vi "ArmTangentPath.vi"(1 "Radius":dbl, 2 "EndPoint":T2, 3 "PathIn":T1[](array[typedef])) -> (0 "PathOut":T1[](array[typedef]))   [LabVIEW 2018]
uses:
  TypeDefs/ArmCoordinate.ctl
  ArgosLib/Path Planning/TypeDefs/Point2D.ctl
  ArgosLib/ArgosLib.lvlib
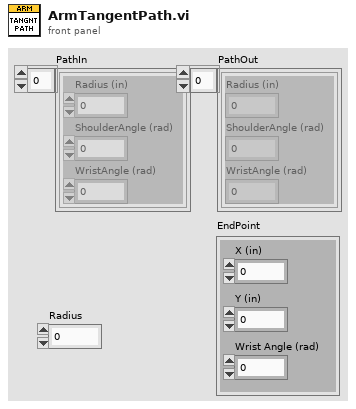
[diagram p1: front panel]
types:
  T1 = typedef "ArmCoordinate.ctl" = cluster{"Radius (in)":dbl, "ShoulderAngle (rad)":dbl, "WristAngle (rad)":dbl}
  T2 = typedef "ArgosLib.lvlib/Point2D.ctl" = cluster{"X (in)":dbl, "Y (in)":dbl, "Wrist Angle (rad)":dbl}
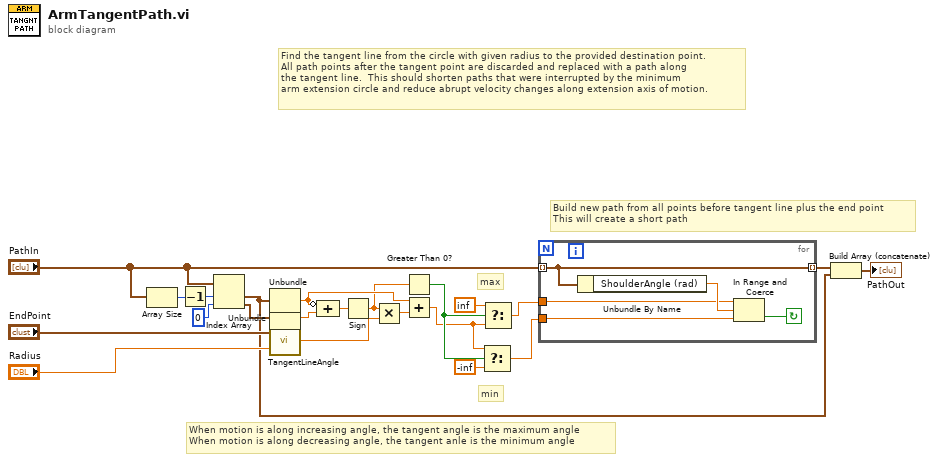
[diagram p0: block diagram]
diagram:
  # "Build new path from all points before tangent line plus the end point\nThis will create a short path"
  # "When motion is along increasing angle, the tangent angle is the maximum angle\nWhen motion is along decreasing angle, the tangent anle is the minimum angle"
  # "Find the tangent line from the circle with given radius to the provided destination point.\nAll path points after the tangent point are discarded and replaced with a path along\nthe tangent line.  This should shorten paths that were interrupted by the minimum\narm extension circle and reduce abrupt velocity changes along extension axis of motion."
  # "max"
  # "min"
  n1 = Array Size(array="PathIn") -> (size(s)=w22:i32)
  n2 = Decrement(x=w22) -> (x-1=w21:i32)
  n3 = Index Array(array="PathIn", index #1=w21, index #2=0 ("index")) -> (element #1=w1:T1, element #2=w6:T1)
  n4 = Unbundle(w1) -> ("ShoulderAngle (rad)"=w16:dbl)  [unwired: 2 out]
  n5 = Unbundle(w6) -> ("ShoulderAngle (rad)"=w19:dbl)  [unwired: 2 out]
  n6 = call "TangentLineAngle.vi"("Radius"="Radius", "DestPoint"="EndPoint") -> ("Tangent Angle Offset (rad)"=w17:dbl)
  n7 = Compound Arithmetic op=ADD(invert w16, w19) -> (w18:dbl)
  n8 = Sign(1:w18) -> (0:w14:dbl)
  n9 = Multiply(x=w14, y=w17) -> (x*y=w15:dbl)
  n10 = Greater Than 0?(x=w14) -> (x > 0?=w13:bool)
  n11 = Add(x=w16, y=w15) -> (x+y=w12:dbl)
  n12 = Select(t=w12, s=w13, f=-inf) -> (s? t:f=w8:dbl)
  n13 = Select(t=inf, s=w13, f=w12) -> (s? t:f=w9:dbl)
  n14 = for {
    tunnel: "PathIn" -> [w23] mode=indexing
    tunnel: w9 -> [w26]
    tunnel: w8 -> [w25]
    tunnel: [w23] -> w7 mode=indexing
    stop <- w24 continue-if-true
    n15 = Unbundle By Name(w23) -> ("ShoulderAngle (rad)"=w27:dbl)
    n16 = In Range and Coerce(upper limit=w26, x=w27, lower limit=w25) -> (In Range?=w24:bool)  [unwired: 1 out]
  }
  n17 = Build Array (concatenate)(w7, w1) -> (→"PathOut":T1[])
